vi "Destroy AO DAQmx Refs.vi"(8 "error in (no error)":errorcluster, 10 "AO":T1 {"Conversion"."ScaleOffset" format="%.3f"; "Conversion"."MinEngUnit" format="%.3f"; "Conversion"."MaxEngUnit" format="%.3f"; "Conversion"."MinSignal" format="%.3f"; "Conversion"."MaxSignal" format="%.3f"}) -> (0 "error out":errorcluster, 2 "AO OUT":T1 {"Conversion"."ScaleOffset" format="%.3f"; "Conversion"."MinEngUnit" format="%.3f"; "Conversion"."MaxEngUnit" format="%.3f"; "Conversion"."MinSignal" format="%.3f"; "Conversion"."MaxSignal" format="%.3f"})   [LabVIEW 2017, in "DAQ.lvclass"]
doc: "Developed by Kevin Thompson\nkevin@thompsonengineering.net\n\nCopyright 2018-2020\nThompson Engineering, LLC"
uses:
  DAQ.lvclass
  DataTypes/TD AO Channel--cluster.ctl
  DataTypes/TD DataValueConversion--cluster.ctl
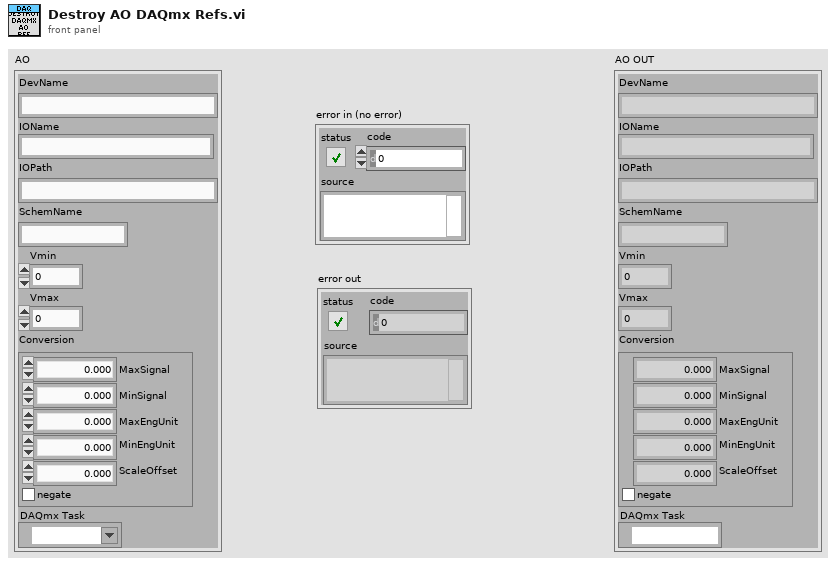
[diagram p1: front panel]
types:
  T1 = typedef "DAQ.lvclass/TD AO Channel--cluster.ctl" = cluster{"DevName":string, "IOName":string, "IOPath":string, "SchemName":string, "Vmin":dbl, "Vmax":dbl, "Conversion":T2, "DAQmx Task":refnum<k21>}
  T2 = typedef "DAQ.lvclass/TD DataValueConversion--cluster.ctl" = cluster{"MaxSignal":dbl, "MinSignal":dbl, "MaxEngUnit":dbl, "MinEngUnit":dbl, "ScaleOffset":dbl, "negate":bool}
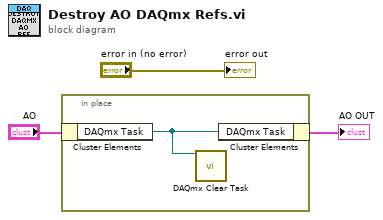
[diagram p0: block diagram]
diagram:
  n1 = in-place {
    n2 = in-place-cluster #1("AO") -> ("DAQmx Task"=w4:refnum<k21>)
    n3 = call <vilib>:"DAQmx Clear Task.vi"("task in"=w4) -> ()  [unwired: 14 in, 1 out]
    n4 = in-place-cluster #1("DAQmx Task"=w4) -> (→"AO OUT":T1)
  }
  "error out" <- "error in (no error)"
